vi "LOGIC_BuildProcName.vi"(11 "Database RefNum in":T1) -> (2 "proc name":string)   [LabVIEW 2016]
uses:
  DBSHAND/private/vis/DatabaseHand_RefNum.ctl
  DBSHAND/private/vis/DatabaseHand_Element_Get(string).vi
  DBSHAND/private/vis/DatabaseHand_Element_Get(bool).vi
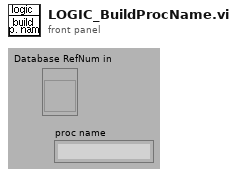
[diagram p1: front panel]
types:
  T1 = typedef "DatabaseHand_RefNum.ctl" = refnum<vi>
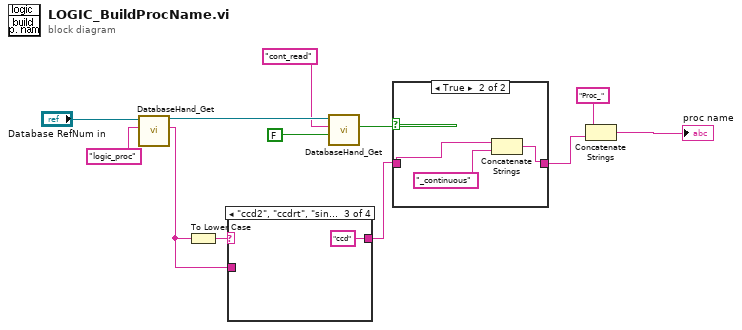
[diagram p0: block diagram]
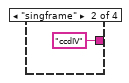
[diagram p3: hidden frame]
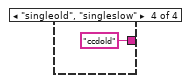
[diagram p4: hidden frame]
diagram:
  n1 = call-poly "DatabaseHand_Get.vi"("name"="logic_proc", "Database RefNum in"="Database RefNum in") -> ("value"=w1:string, "Database RefNum out"=w10:T1)  [unwired: 3 in, 5 out]
  n2 = To Lower Case(string=w1) -> (all lower case string=w2:string)
  n3 = case shown="\"ccd2\", \"ccdrt\", \"single\"" w2 {
    tunnel: [w13 "ccdIV" "ccd" "ccdold"] -> w3
    tunnel: w1 -> [w13 _ _ _]
    frame Default {
    }
    frame "singframe" {
    }
    frame "ccd2", "ccdrt", "single" {
    }
    frame "singleold", "singleslow" {
    }
  }
  n4 = call-poly "DatabaseHand_Get.vi"("default value"=FALSE, "name"="cont_read", "Database RefNum in"=w10) -> ("value"=w7:bool)  [unwired: 2 in, 6 out]
  n5 = case shown="True" w7 {
    tunnel: w3 -> [w17 w20]
    tunnel: [w17 w18] -> w6
    frame False {
    }
    frame True {
      n6 = Concatenate Strings(w20, "_continuous" ("string")) -> (w18:string)
    }
  }
  n7 = Concatenate Strings("Proc_", w6) -> (→"proc name":string)
